vi "SSH Close.vi"(8 "Error In":errorcluster, 11 "SSH Session":refnum<k1>) -> (0 "Error Out":errorcluster)   [LabVIEW 2019, in "LMH-LINX.lvlib"]
uses:
  <vilib>/MakerHub/LINX/LMH-LINX.lvlib
  E:/lv2019/dist/vi.lib/MakerHub/LINX/Resources/Renci.SshNet.dll
  Resources/Renci.SshNet.dll
  <vilib>/MakerHub/LINX/Private/Utilties/SSH/SSH Unix Session Op.ctl
  usr/lib/system/libsystem_c.dylib
  libc.so.6
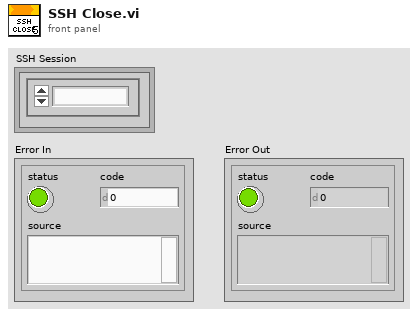
[diagram p1: front panel]
types:
  T1 = typedef "LMH-LINX.lvlib/SSH Unix Session Op.ctl" = enum16{"New", "Get", "Delete"}
  T2 = typedef "LMH-LINX.lvlib/SSH Unix Session Info.ctl" = cluster{"PID":i32, "Read FD":i32, "Write FD":i32, "Error FD":i32}
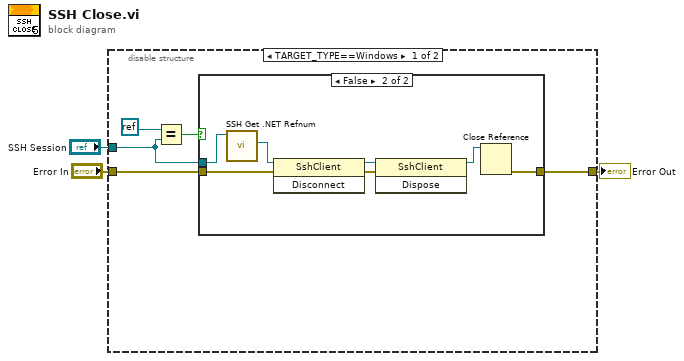
[diagram p0: block diagram]
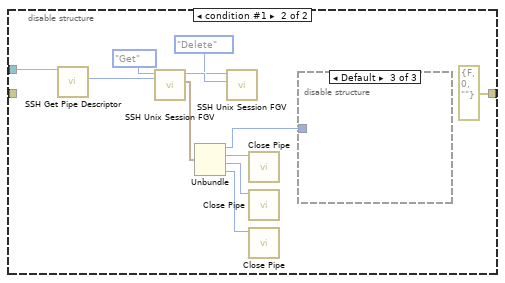
[diagram p3: hidden frame]
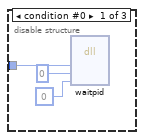
[diagram p4: hidden frame]
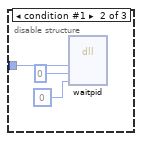
[diagram p5: hidden frame]
diagram:
  n1 = disable-structure shown="TARGET_TYPE==Windows" {
    disable-tunnel: "Error In" -> [w8 _]
    disable-tunnel: [w7 errorcluster {"status"=FALSE, "code"=0, "source"=""} ("Error Out")] -> w2
    disable-tunnel: "SSH Session" -> [w4 w27]
    frame condition #0 (active) {
      n2 = Equal?(x=refnum<k0> refnum, y=w4) -> (x = y?=w5:bool)
      n3 = case shown="False" w5 {
        tunnel: w8 -> [w9 w14]
        tunnel: [w9 w13] -> w7
        tunnel: w4 -> [_ w11]
        frame True {
        }
        frame False {
          n4 = call <vilib>:"SSH Get .NET Refnum.vi"("SSH Session"=w11) -> ("SSH .NET Refnum"=w10:refnum<k24>)  [unwired: 8 in, 2 out]
          n5 = invoke class="SshClient" method="Disconnect"(reference=w10, error in=w14) -> (reference out=w15:refnum<k24>, error out=w16:errorcluster)  [unwired: 1 in, 1 out]
          n6 = invoke class="SshClient" method="Dispose"(reference=w15, error in=w16) -> (reference out=w12:refnum<k24>)  [unwired: 1 in, 2 out]
          n7 = Close Reference(reference=w12) -> (error out=w13:errorcluster)  [unwired: 1 in]
        }
      }
    }
    frame condition #1 {
      n8 = call <vilib>:"SSH Get Pipe Descriptor.vi"("SSH Session"=w27) -> ("SSH Pipe Descriptor"=w26:i32)  [unwired: 8 in, 2 out]
      n9 = call <vilib>:"SSH Unix Session FGV.vi"("Session In"=w26, "Operation"=SSH_Unix_Session_Op."Get") -> ("info in"=w20:T2, "Session Out"=w19:i32)  [unwired: 8 in]
      n10 = Unbundle(w20) -> ("PID"=w21:i32, "Read FD"=w24:i32, "Write FD"=w23:i32, "Error FD"=w22:i32)
      n11 = call <vilib>:"SSH Unix Session FGV.vi"("Session In"=w19, "Operation"=SSH_Unix_Session_Op."Delete") -> ()  [unwired: 8 in, 2 out]
      n12 = call <vilib>:"Close Pipe.vi"("file descriptor"=w24) -> ()  [unwired: 5 in, 2 out]
      n13 = call <vilib>:"Close Pipe.vi"("file descriptor"=w23) -> ()  [unwired: 5 in, 2 out]
      n14 = call <vilib>:"Close Pipe.vi"("file descriptor"=w22) -> ()  [unwired: 5 in, 2 out]
      n15 = disable-structure shown="Default" {
        disable-tunnel: w21 -> [w30 w33 _]
        frame condition #0 {
          n16 = dll-call lib="usr/lib/system/libsystem_c.dylib" fn="waitpid"("pid"=w30, "stat"=0, "options"=0) -> ()  [unwired: 7 in, 2 out]
        }
        frame condition #1 {
          n17 = dll-call lib="libc.so.6" fn="waitpid"("pid"=w33, "status"=0, "options"=0) -> ()  [unwired: 7 in, 2 out]
        }
        frame condition #2 (active) {
        }
      }
    }
  }
  "Error Out" <- w2
